vi "ROI entry screen-LBox filter update rows.vi"(8 "error in (no error)":errorcluster, 9 "Show All":bool, 10 "Stop Plane":i32, 11 "Start Plane":i32) -> (0 "error out":errorcluster, 3 "Array":bool[](array[boolean]))   [LabVIEW 2020]
uses:
  Globals/gl_ROI Entry UI globals.vi
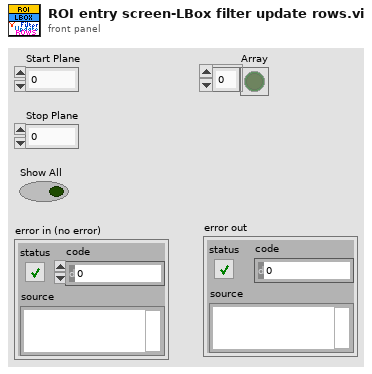
[diagram p1: front panel]
types:
  T1 = typedef "ROI entry screen ctrl refs cluster.ctl" = cluster{"Done button":refnum<vi>, "Imaging button":refnum<vi>, "Acquisition button":refnum<vi>, "Scan dwell time per pixel (us)":refnum<vi>, "# of planes":refnum<vi>, "Zoom Ctrl":refnum<vi>, "Equal size":refnum<vi>, "Channel":refnum<vi>, "Image Display":refnum<vi>, "Z-Plane Selector":refnum<vi>, "Number of lines left":refnum<vi>, "Z-stack folder path":refnum<vi>, "POI Density":refnum<vi>, "Arb Plane Entry":refnum<vi>, "Whole Plane":refnum<vi>, "Line Mode":refnum<vi>, "Clear Last":refnum<vi>, "Clear All":refnum<vi>, "Delete Lines":refnum<vi>, "Trial Length (sec)":refnum<vi>, "Palette Type":refnum<vi>, "Intensity slider":refnum<vi>, "# POI":refnum<vi>, "Max Z Proj":refnum<vi>, "Zplane ind":refnum<vi>, "Wavelength (nm)":refnum<vi>, "Number of Trials":refnum<vi>, "Funct stim.trig.enable":refnum<vi>, "Funct stim.trig.delay (s)":refnum<vi>, "Line Mode":refnum<vi>, "Step size (µm)":refnum<vi>, "ROI move mode":refnum<vi>, "Cool-down time (s)":refnum<vi>, "Enable cool-down time":refnum<vi>, "Motor Z ind. (um)":refnum<vi>, "AOL Z ind. (um)":refnum<vi>, "Load Reference Image":refnum<vi>, "Rel.  Res.":refnum<vi>, "ROI LIST":refnum<vi>, "Show All":refnum<vi>, "ROI Type":refnum<vi>, "Start Plane":refnum<vi>, "Stop Plane":refnum<vi>, "Offset ROI":refnum<vi>, "Tab Control":refnum<vi>, "Laser Power(%)":refnum<vi>, "Cycle rate":refnum<vi>, "FOV (Ind.)":refnum<vi>, "Frame Size (Ind.)":refnum<vi>, "Resolution (Ind.)":refnum<vi>, "Pixel Density (Ind)":refnum<vi>, "Laser Power (Ind.)":refnum<vi>, "Dwell Time (Ind.)":refnum<vi>, "Adj MC":refnum<vi>}
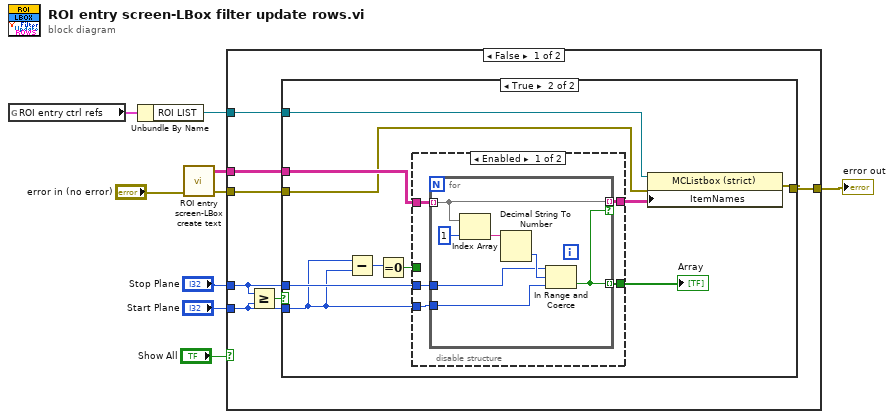
[diagram p0: block diagram]
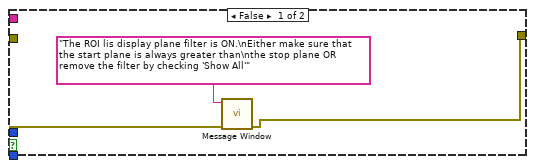
[diagram p2: hidden frame]
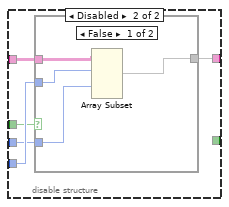
[diagram p3: hidden frame]
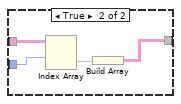
[diagram p4: hidden frame]
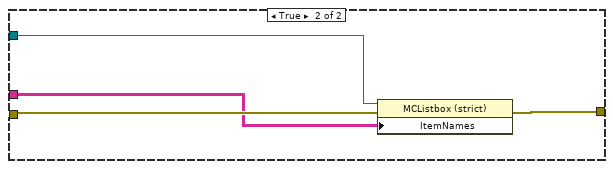
[diagram p5: hidden frame]
diagram:
  n1 = global read "gl_ROI Entry UI globals.vi" "ROI entry ctrl refs"() -> (w2:T1)
  n2 = Unbundle By Name(w2) -> ("ROI LIST"=w1:refnum<vi>)
  n3 = call "ROI entry screen-LBox create text.vi"("error in (no error)"="error in (no error)") -> ("error out"=w4:errorcluster, "Array"=w3:string[][])  [unwired: 9 in]
  n4 = case shown="False" "Show All" {
    tunnel: w4 -> [w11 w58]
    tunnel: "Start Plane" -> [w15 _]
    tunnel: "Stop Plane" -> [w16 _]
    tunnel: [w13 w57] -> w6
    tunnel: w3 -> [w12 w56]
    tunnel: w1 -> [w10 w55]
    frame False {
      n5 = Greater Or Equal?(x=w16, y=w15) -> (x >= y?=w14:bool)
      n6 = case shown="True" w14 {
        tunnel: w10 -> [_ w23]
        tunnel: w15 -> [_ w24]
        tunnel: w16 -> [_ w28]
        tunnel: w11 -> [w19 w20]
        tunnel: [w18 w22] -> w13
        tunnel: w12 -> [_ w21]
        frame False {
          n7 = call "Message Window.vi"("error in (no error)"=w19, "Message string"="The ROI lis display plane filter is ON.\nEither make sure that the start plane is always greater than\nthe stop plane OR remove the filter by checking 'Show All'") -> ("error out (no error)"=w18:errorcluster)  [unwired: 9 in]
        }
        frame True {
          n8 = Subtract(x=w24, y=w24) -> (x-y=w27:i32)
          n9 = Equal To 0?(x=w27) -> (x = 0?=w26:bool)
          n10 = disable-structure shown="Enabled" {
            disable-tunnel: w21 -> [w34 w46]
            disable-tunnel: w24 -> [w33 w45]
            disable-tunnel: w28 -> [w32 w43]
            disable-tunnel: [w31 w42] -> w29
            disable-tunnel: w26 -> [_ w44]
            disable-tunnel: [w30 _] -> w25
            frame Enabled {
              n11 = for {
                tunnel: w34 -> [w38] mode=indexing
                tunnel: w33 -> [w35]
                tunnel: w32 -> [w36]
                tunnel: [w38] -> w31 mode=indexing if=w37
                tunnel: [w37] -> w30 mode=indexing
                n12 = Index Array(array=w38, index=1) -> (element=w40:string)
                n13 = Decimal String To Number(string=w40) -> (number=w39:i32)  [unwired: 2 in, 1 out]
                n14 = In Range and Coerce(upper limit=w36, x=w39, lower limit=w35) -> (In Range?=w37:bool)  [unwired: 1 out]
              }
            }
            frame Disabled {
              n15 = case shown="False" w44 {
                tunnel: w46 -> [w50 w54]
                tunnel: w45 -> [w49 w53]
                tunnel: w43 -> [w48 _]
                tunnel: [w47 w51] -> w42
                frame False {
                  n16 = Array Subset(array=w50, index (row)=w49, index (col)=w48) -> (w47:string[][])  [unwired: 2 in]
                }
                frame True {
                  n17 = Index Array(array=w54, index (row)=w53) -> (element=w52:string[])  [unwired: 1 in]
                  n18 = Build Array(w52) -> (w51:string[][])
                }
              }
            }
          }
          "Array" <- w25
          n19 = property class="MCListbox (strict)"(reference=w23, error in=w20, "ItemNames"=w29) -> (error out=w22:errorcluster)  [unwired: 1 out]
        }
      }
    }
    frame True {
      n20 = property class="MCListbox (strict)"(reference=w55, error in=w58, "ItemNames"=w56) -> (error out=w57:errorcluster)  [unwired: 1 out]
    }
  }
  "error out" <- w6
